vi "setFirstTimestamp.vi"(8 "error in (no error)":errorcluster, 11 "PeriodicWave in":refnum<class "PeriodicWave.lvclass">) -> (0 "error out":errorcluster, 3 "PeriodicWave out":refnum<class "PeriodicWave.lvclass">)   [LabVIEW 2015, in "PeriodicWave.lvclass"]
uses:
  PeriodicWave.lvclass
  PeriodicWave.lvclass/PeriodicWave.ctl
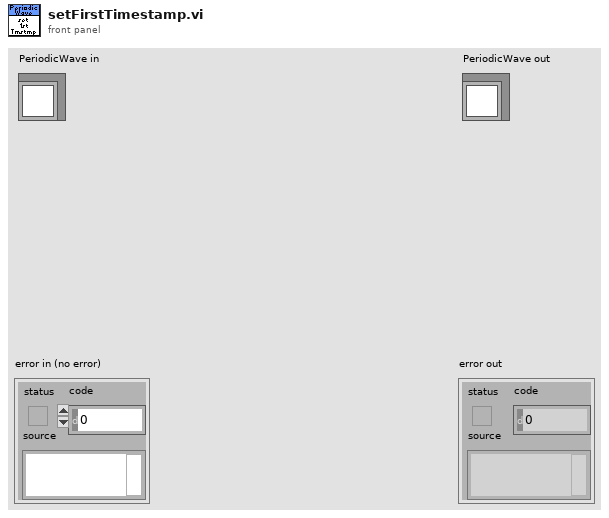
[diagram p1: front panel]
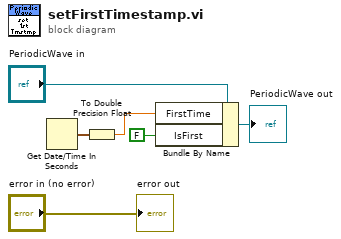
[diagram p0: block diagram]
diagram:
  n1 = Get Date/Time In Seconds() -> (seconds since 1Jan1904=w5:timestamp)
  n2 = To Double Precision Float(number=w5) -> (double precision float=w4:dbl)
  n3 = Bundle By Name(cluster="PeriodicWave in", "FirstTime"=w4, "IsFirst"=FALSE) -> (→"PeriodicWave out":refnum<class "PeriodicWave.lvclass">)
  "error out" <- "error in (no error)"
